vi "ReadTablesWithinSpreadsheet_BackUp_ver2.vi"(8 "Error In":errorcluster, 11 "all rows":string[][](array[string])=[["#param1", "param2", "param3", "param4", "", "", "", "", "", ""], ["1.00", "1.20", "1.30", "1.40", "", "", "", "", "", ""], ["2.00", "2.20", "2.30", "2.40", "", "", "", "", "", ""], ["3.00", "3.20", "3.30", "3.40", "", "", "", "", "", ""], ["4.00", "4.20", "4.30", "4.40", "", "", "", "", "", ""], ["", "", "", "", "", "", "", "", "", ""], ["", "", "", "", "", "", "", "", "", ""], ["#A", "B", "C", "D", "E", "F", "G", "H", "I", "J"], ["0,372", "0,372", "0,372", "0,372", "0,372", "0,372", "0,372", "0,372", "0,372", "0,372"], ["0,735", "0,735", "0,735", "0,735", "0,735", "0,735", "0,735", "0,735", "0,735", "0,735"], ["0,731", "0,731", "0,731", "0,731", "0,731", "0,731", "0,731", "0,731", "0,731", "0,731"], ["0,139", "0,139", "0,139", "0,139", "0,139", "0,139", "0,139", "0,139", "0,139", "0,139"], ["0,692", "0,692", "0,692", "0,692", "0,692", "0,692", "0,692", "0,692", "0,692", "0,692"], ["0,681", "0,681", "0,681", "0,681", "0,681", "0,681", "0,681", "0,681", "0,681", "0,681"], ["0,918", "0,918", "0,918", "0,918", "0,918", "0,918", "0,918", "0,918", "0,918", "0,918"], ["0,872", "0,872", "0,872", "0,872", "0,872", "0,872", "0,872", "0,872", "0,872", "0,872"], ["0,797", "0,797", "0,797", "0,797", "0,797", "0,797", "0,797", "0,797", "0,797", "0,797"], ["0,041", "0,041", "0,041", "0,041", "0,041", "0,041", "0,041", "0,041", "0,041", "0,041"], ["", "", "", "", "", "", "", "", "", ""], ["", "", "", "", "", "", "", "", "", ""], ["", "", "", "", "", "", "", "", "", ""], ["", "", "", "", "", "", "", "", "", ""], ["", "", "", "", "", "", "", "", "", ""], ["#Z", "Y", "X", "W", "V", "U", "T", "S", "R", "Q"], ["0,372", "0,372", "0,372", "0,372", "0,372", "0,372", "0,372", "0,372", "0,372", "0,372"], ["0,735", "0,735", "0,735", "0,735", "0,735", "0,735", "0,735", "0,735", "0,735", "0,735"], ["0,731", "0,731", "0,731", "0,731", "0,731", "0,731", "0,731", "0,731", "0,731", "0,731"], ["", "", "", "", "", "", "", "", "", ""], ["", "", "", "", "", "", "", "", "", ""], ["#Z", "Y", "X", "W", "V", "U", "T", "S", "R", "Q"], ["0,372", "0,372", "0,372", "0,372", "0,372", "0,372", "0,372", "0,372", "0,372", "0,372"], ["0,735", "0,735", "0,735", "0,735", "0,735", "0,735", "0,735", "0,735", "0,735", "0,735"], ["0,731", "0,731", "0,731", "0,731", "0,731", "0,731", "0,731", "0,731", "0,731", "0,731"], ["0,372", "0,372", "0,372", "0,372", "0,372", "0,372", "0,372", "0,372", "0,372", "0,372"], ["0,735", "0,735", "0,735", "0,735", "0,735", "0,735", "0,735", "0,735", "0,735", "0,735"], ["0,731", "0,731", "0,731", "0,731", "0,731", "0,731", "0,731", "0,731", "0,731", "0,731"], ["0,372", "0,372", "0,372", "0,372", "0,372", "0,372", "0,372", "0,372", "0,372", "0,372"], ["0,735", "0,735", "0,735", "0,735", "0,735", "0,735", "0,735", "0,735", "0,735", "0,735"], ["0,731", "0,731", "0,731", "0,731", "0,731", "0,731", "0,731", "0,731", "0,731", "0,731"], ["0,372", "0,372", "0,372", "0,372", "0,372", "0,372", "0,372", "0,372", "0,372", "0,372"], ["0,735", "0,735", "0,735", "0,735", "0,735", "0,735", "0,735", "0,735", "0,735", "0,735"], ["0,731", "0,731", "0,731", "0,731", "0,731", "0,731", "0,731", "0,731", "0,731", "0,731"], ["0,372", "0,372", "0,372", "0,372", "0,372", "0,372", "0,372", "0,372", "0,372", "0,372"], ["0,735", "0,735", "0,735", "0,735", "0,735", "0,735", "0,735", "0,735", "0,735", "0,735"], ["0,731", "0,731", "0,731", "0,731", "0,731", "0,731", "0,731", "0,731", "0,731", "0,731"], ["0,372", "0,372", "0,372", "0,372", "0,372", "0,372", "0,372", "0,372", "0,372", "0,372"], ["0,735", "0,735", "0,735", "0,735", "0,735", "0,735", "0,735", "0,735", "0,735", "0,735"], ["0,731", "0,731", "0,731", "0,731", "0,731", "0,731", "0,731", "0,731", "0,731", "0,731"], ["0,372", "0,372", "0,372", "0,372", "0,372", "0,372", "0,372", "0,372", "0,372", "0,372"], ["0,735", "0,735", "0,735", "0,735", "0,735", "0,735", "0,735", "0,735", "0,735", "0,735"], ["0,731", "0,731", "0,731", "0,731", "0,731", "0,731", "0,731", "0,731", "0,731", "0,731"], ["0,372", "0,372", "0,372", "0,372", "0,372", "0,372", "0,372", "0,372", "0,372", "0,372"], ["0,735", "0,735", "0,735", "0,735", "0,735", "0,735", "0,735", "0,735", "0,735", "0,735"], ["0,731", "0,731", "0,731", "0,731", "0,731", "0,731", "0,731", "0,731", "0,731", "0,731"], ["0,372", "0,372", "0,372", "0,372", "0,372", "0,372", "0,372", "0,372", "0,372", "0,372"], ["0,735", "0,735", "0,735", "0,735", "0,735", "0,735", "0,735", "0,735", "0,735", "0,735"], ["0,731", "0,731", "0,731", "0,731", "0,731", "0,731", "0,731", "0,731", "0,731", "0,731"], ["0,372", "0,372", "0,372", "0,372", "0,372", "0,372", "0,372", "0,372", "0,372", "0,372"], ["0,735", "0,735", "0,735", "0,735", "0,735", "0,735", "0,735", "0,735", "0,735", "0,735"], ["0,731", "0,731", "0,731", "0,731", "0,731", "0,731", "0,731", "0,731", "0,731", "0,731"], ["0,372", "0,372", "0,372", "0,372", "0,372", "0,372", "0,372", "0,372", "0,372", "0,372"], ["0,735", "0,735", "0,735", "0,735", "0,735", "0,735", "0,735", "0,735", "0,735", "0,735"], ["0,731", "0,731", "0,731", "0,731", "0,731", "0,731", "0,731", "0,731", "0,731", "0,731"], ["0,372", "0,372", "0,372", "0,372", "0,372", "0,372", "0,372", "0,372", "0,372", "0,372"], ["0,735", "0,735", "0,735", "0,735", "0,735", "0,735", "0,735", "0,735", "0,735", "0,735"], ["0,731", "0,731", "0,731", "0,731", "0,731", "0,731", "0,731", "0,731", "0,731", "0,731"], ["0,372", "0,372", "0,372", "0,372", "0,372", "0,372", "0,372", "0,372", "0,372", "0,372"], ["0,735", "0,735", "0,735", "0,735", "0,735", "0,735", "0,735", "0,735", "0,735", "0,735"], ["0,731", "0,731", "0,731", "0,731", "0,731", "0,731", "0,731", "0,731", "0,731", "0,731"], ["0,372", "0,372", "0,372", "0,372", "0,372", "0,372", "0,372", "0,372", "0,372", "0,372"], ["0,735", "0,735", "0,735", "0,735", "0,735", "0,735", "0,735", "0,735", "0,735", "0,735"], ["0,731", "0,731", "0,731", "0,731", "0,731", "0,731", "0,731", "0,731", "0,731", "0,731"], ["0,372", "0,372", "0,372", "0,372", "0,372", "0,372", "0,372", "0,372", "0,372", "0,372"], ["0,735", "0,735", "0,735", "0,735", "0,735", "0,735", "0,735", "0,735", "0,735", "0,735"], ["0,731", "0,731", "0,731", "0,731", "0,731", "0,731", "0,731", "0,731", "0,731", "0,731"], ["0,372", "0,372", "0,372", "0,372", "0,372", "0,372", "0,372", "0,372", "0,372", "0,372"], ["0,735", "0,735", "0,735", "0,735", "0,735", "0,735", "0,735", "0,735", "0,735", "0,735"], ["0,731", "0,731", "0,731", "0,731", "0,731", "0,731", "0,731", "0,731", "0,731", "0,731"], ["0,372", "0,372", "0,372", "0,372", "0,372", "0,372", "0,372", "0,372", "0,372", "0,372"], ["0,735", "0,735", "0,735", "0,735", "0,735", "0,735", "0,735", "0,735", "0,735", "0,735"], ["0,731", "0,731", "0,731", "0,731", "0,731", "0,731", "0,731", "0,731", "0,731", "0,731"], ["0,372", "0,372", "0,372", "0,372", "0,372", "0,372", "0,372", "0,372", "0,372", "0,372"], ["0,735", "0,735", "0,735", "0,735", "0,735", "0,735", "0,735", "0,735", "0,735", "0,735"], ["0,731", "0,731", "0,731", "0,731", "0,731", "0,731", "0,731", "0,731", "0,731", "0,731"], ["0,372", "0,372", "0,372", "0,372", "0,372", "0,372", "0,372", "0,372", "0,372", "0,372"], ["0,735", "0,735", "0,735", "0,735", "0,735", "0,735", "0,735", "0,735", "0,735", "0,735"], ["0,731", "0,731", "0,731", "0,731", "0,731", "0,731", "0,731", "0,731", "0,731", "0,731"], ["0,372", "0,372", "0,372", "0,372", "0,372", "0,372", "0,372", "0,372", "0,372", "0,372"], ["0,735", "0,735", "0,735", "0,735", "0,735", "0,735", "0,735", "0,735", "0,735", "0,735"], ["0,731", "0,731", "0,731", "0,731", "0,731", "0,731", "0,731", "0,731", "0,731", "0,731"], ["0,372", "0,372", "0,372", "0,372", "0,372", "0,372", "0,372", "0,372", "0,372", "0,372"], ["0,735", "0,735", "0,735", "0,735", "0,735", "0,735", "0,735", "0,735", "0,735", "0,735"], ["0,731", "0,731", "0,731", "0,731", "0,731", "0,731", "0,731", "0,731", "0,731", "0,731"], ["0,372", "0,372", "0,372", "0,372", "0,372", "0,372", "0,372", "0,372", "0,372", "0,372"], ["0,735", "0,735", "0,735", "0,735", "0,735", "0,735", "0,735", "0,735", "0,735", "0,735"], ["0,731", "0,731", "0,731", "0,731", "0,731", "0,731", "0,731", "0,731", "0,731", "0,731"], ["0,372", "0,372", "0,372", "0,372", "0,372", "0,372", "0,372", "0,372", "0,372", "0,372"], ["0,735", "0,735", "0,735", "0,735", "0,735", "0,735", "0,735", "0,735", "0,735", "0,735"], ["0,731", "0,731", "0,731", "0,731", "0,731", "0,731", "0,731", "0,731", "0,731", "0,731"], ["0,372", "0,372", "0,372", "0,372", "0,372", "0,372", "0,372", "0,372", "0,372", "0,372"], ["0,735", "0,735", "0,735", "0,735", "0,735", "0,735", "0,735", "0,735", "0,735", "0,735"], ["0,999", "0,888", "0,731", "0,731", "0,731", "0,731", "0,731", "0,731", "0,731", "0,731"], ["", "", "", "", "", "", "", "", "", ""], ["", "", "", "", "", "", "", "", "", ""], ["", "", "", "", "", "", "", "", "", ""]]) -> (0 "Error Out":errorcluster, 3 "Of Data-Tables (Out)":T1[](array[typedef]))   [LabVIEW 2014]
uses:
  ReadTablesWithinSpreadsheet_ver13/Table_Cluster_Control.ctl
  <userlib>/_OpenG.lib/array/array.llb/Filter 1D Array with Scalar (String)__ogtk.vi
  <userlib>/_OpenG.lib/array/array.llb/Empty 1D Array (String)__ogtk.vi
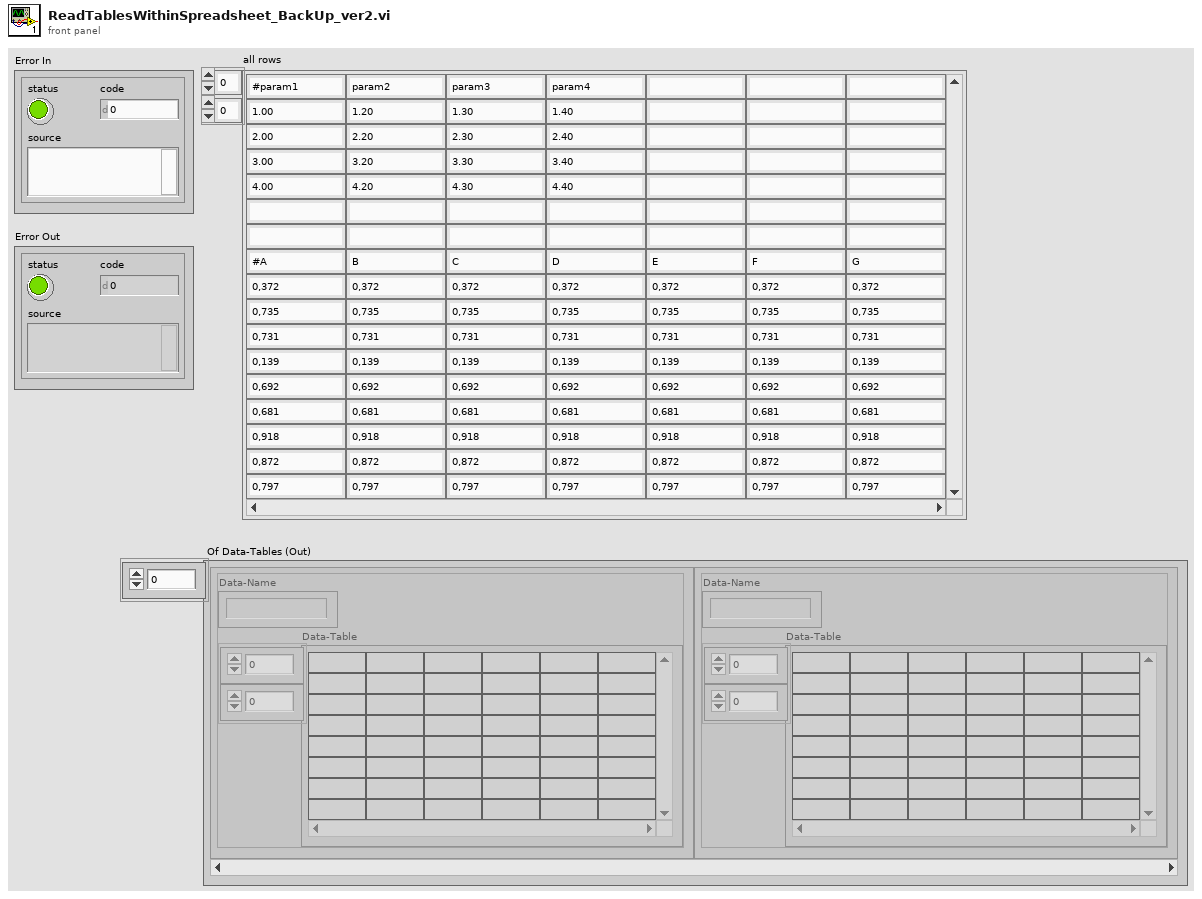
[diagram p1: front panel]
types:
  T1 = typedef "Table_Cluster_Control.ctl" = cluster{"Data-Name":string, "Data-Table":string[][]}
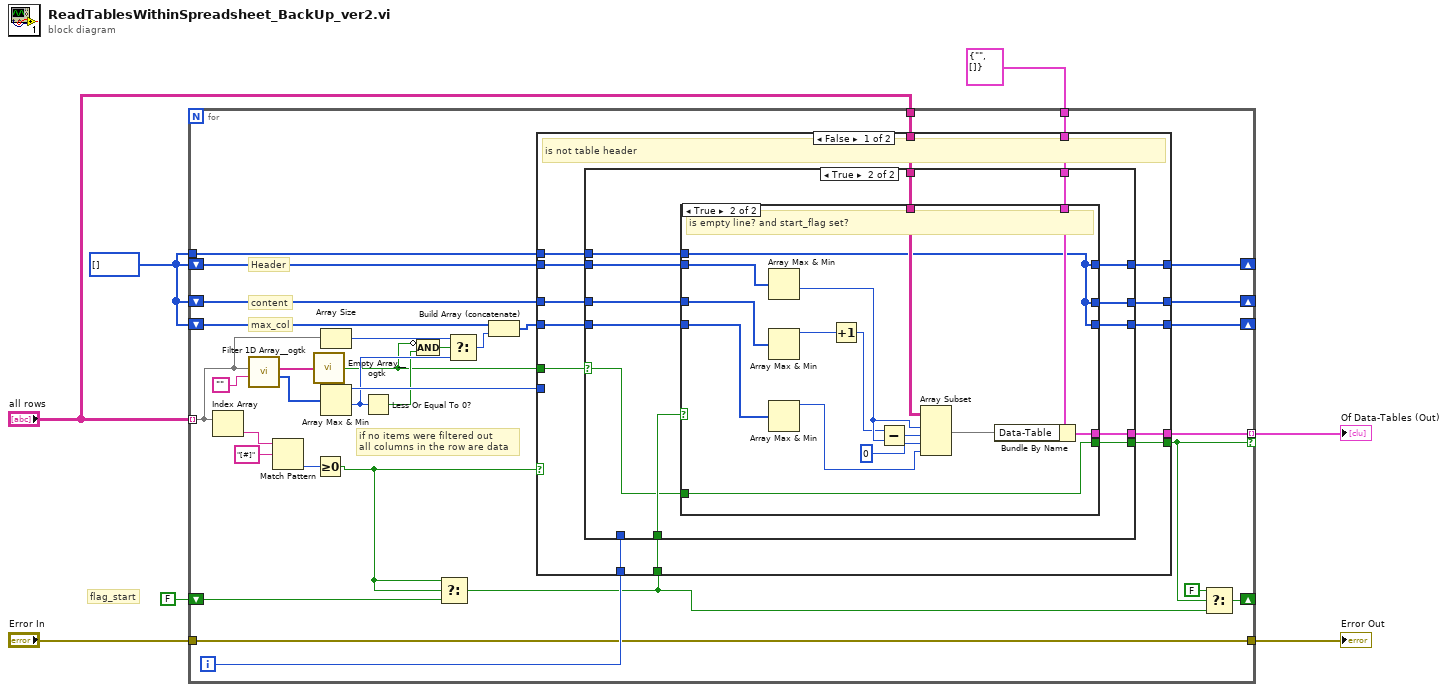
[diagram p0: block diagram]
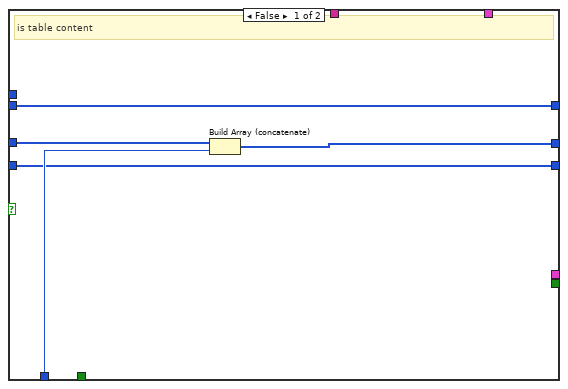
[diagram p2: hidden frame]
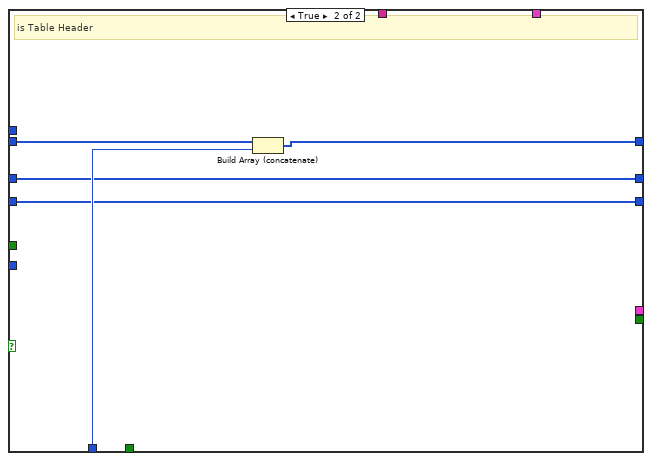
[diagram p4: hidden frame]
diagram:
  w7 = i32[] [] ("filtered item indices")
  # "flag_start"
  n1 = for {
    tunnel: "all rows" -> [w15] mode=indexing
    shift-right: [w34] -> _
    shift-left: w7 -> [w35]
    shift-right: [w30] -> _
    shift-left: w7 -> [w32]
    shift-right: [w31] -> _
    shift-left: w7 -> [w28]
    tunnel: "all rows" -> [w29]
    tunnel: w7 -> [w26]
    tunnel: T1 {"Data-Name"="", "Data-Table"=[]} -> [w25]
    tunnel: [w24] -> w5 mode=indexing if=w21
    shift-right: [w20] -> _
    shift-left: FALSE -> [w22]
    tunnel: "Error In" -> [w14]
    tunnel: [w14] -> w1
    i -> [w33]
    # "if no items were filtered out\nall columns in the row are data"
    # "max_col"
    # "content"
    # "Header"
    n2 = Index Array(array=w15) -> (element=w36:string)  [unwired: 1 in]
    n3 = call-poly <userlib>:"Filter 1D Array__ogtk.vi"("items to filter"="", "array"=w15) -> ("filtered item indices"=w40:i32[], "filtered array"=w17:string[])  [unwired: 4 in]
    n4 = Match Pattern(string=w36, regular expression="[#]") -> (offset past match=w39:i32)  [unwired: 1 in, 3 out]
    n5 = call-poly <userlib>:"Empty Array__ogtk.vi"("Array"=w17) -> ("Empty Array?"=w9:bool)  [unwired: 8 in]
    n6 = Greater Or Equal To 0?(x=w39) -> (x >= 0?=w19:bool)
    n7 = Array Size(array=w15) -> (size(s)=w16:i32)
    n8 = Array Max & Min(array=w40) -> (max value=w13:i32, min value=w12:i32)  [unwired: 2 out]
    n9 = Less Or Equal To 0?(x=w12) -> (x <= 0?=w10:bool)
    n10 = Compound Arithmetic op=AND(invert w9, w10) -> (w8:bool)
    n11 = Select(t=w19, s=w19, f=w22) -> (s? t:f=w18:bool)
    n12 = Select(t=w16, s=w8, f=w12) -> (s? t:f=w11:i32)
    n13 = Build Array (concatenate)(w28, w11) -> (w27:i32[])
    n14 = case shown="False" w19 {
      tunnel: w9 -> [w54 _]
      tunnel: w35 -> [w47 w95]
      tunnel: [w48 w94] -> w34
      tunnel: w33 -> [w51 w93]
      tunnel: w32 -> [w53 w91]
      tunnel: w27 -> [w52 w92]
      tunnel: [w50 w92] -> w31
      tunnel: [w49 w91] -> w30
      tunnel: w29 -> [w46 _]
      tunnel: w26 -> [w45 _]
      tunnel: w25 -> [w44 _]
      tunnel: [w43 _] -> w24
      tunnel: [w42 _] -> w21
      tunnel: w18 -> [w41 _]
      tunnel: w13 -> [_ _]
      frame False {
        # "is not table header"
        n15 = case shown="True" w54 {
          selector: w54 -> [_ w60]
          tunnel: w53 -> [w59 w71]
          tunnel: w52 -> [w56 w69]
          tunnel: w51 -> [w58 _]
          tunnel: [w56 w63] -> w50
          tunnel: [w57 w64] -> w49
          tunnel: [w55 w65] -> w48
          tunnel: w47 -> [w55 w72]
          tunnel: w46 -> [_ w70]
          tunnel: w45 -> [_ w62]
          tunnel: w44 -> [_ w68]
          tunnel: [_ w67] -> w43
          tunnel: [_ w61] -> w42
          tunnel: w41 -> [_ w66]
          frame False {
            # "is table content"
            n16 = Build Array (concatenate)(w59, w58) -> (w57:i32[])
          }
          frame True {
            n17 = case shown="True" w66 {
              tunnel: w72 -> [w75 w90]
              tunnel: w71 -> [w74 w89]
              tunnel: w70 -> [_ w88]
              tunnel: w69 -> [w73 w85]
              tunnel: w68 -> [_ w82]
              tunnel: [_ w81] -> w67
              tunnel: [w75 w80] -> w65
              tunnel: [w74 w80] -> w64
              tunnel: [w73 w80] -> w63
              tunnel: w62 -> [_ w80]
              tunnel: [_ w79] -> w61
              tunnel: w60 -> [_ w79]
              frame False {
                # "do nothing"
              }
              frame True {
                # "is empty line? and start_flag set?"
                n18 = Array Max & Min(array=w90) -> (min value=w78:i32)  [unwired: 3 out]
                n19 = Array Max & Min(array=w89) -> (max value=w77:i32)  [unwired: 3 out]
                n20 = Array Max & Min(array=w85) -> (max value=w84:i32)  [unwired: 3 out]
                n21 = Increment(x=w77) -> (x+1=w76:i32)
                n22 = Subtract(x=w76, y=w78) -> (x-y=w87:i32)
                n23 = Array Subset(array=w88, index (row)=w78, length (row)=w87, index (col)=0 ("index"), length (col)=w84) -> (w83:string[][])
                n24 = Bundle By Name(cluster=w82, "Data-Table"=w83) -> (w81:T1)
              }
            }
          }
        }
      }
      frame True {
        # "is Table Header"
        n25 = Build Array (concatenate)(w95, w93) -> (w94:i32[])
      }
    }
    n26 = Select(t=FALSE, s=w21, f=w18) -> (s? t:f=w20:bool)
  }
  "Of Data-Tables (Out)" <- w5
  "Error Out" <- w1
